vi "Retrieve Current Sample Data.vi"(8 "error in (no error)":errorcluster) -> (0 "error out":errorcluster, 1 "Last Sample":u32[](array[numeric]), 2 "Encoder Out":i32, 3 "Last Sample No.":u32, 4 "Partial Data":bool, 5 "nSamples":u32)   [LabVIEW 2015, in "Tool Module.lvlib"]
uses:
  Tool Module.lvlib
  ToolModGLOB.vi
  Tool Interface/Tool Interface.lvlib
  Tool Config/Tool Cfg.lvlib
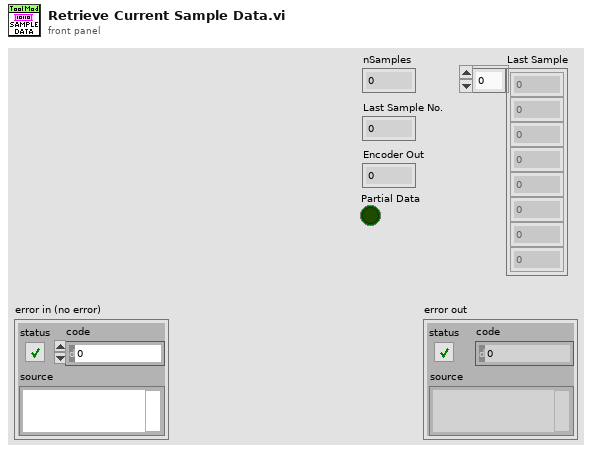
[diagram p1: front panel]
types:
  T1 = typedef "_Data Stream Fmt Params Cluster--typedef.ctl" = cluster{"Samples per Block":i32, "Raw Data Status Len":i32, "Fltr Data Status Len":i32}
  T2 = typedef "Tool Cfg.lvlib/_Tool Operation Config Cluster--typedef.ctl" = cluster{"Use Tool Cfg":bool, "Use Tool Cal":bool, "Fake Data?":bool, "Mode":i16, "Array Subset Length":i16, "nArrays to Read":i16, "Full Array Read Length":i16, "nSubarrays/Sensor":i16}
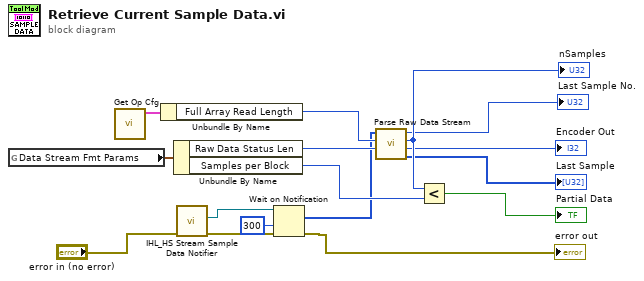
[diagram p0: block diagram]
diagram:
  n1 = global read "ToolModGLOB.vi" "Data Stream Fmt Params"() -> (w11:T1)
  n2 = call "Get Op Cfg.vi"() -> ("Tool Operation Config"=w13:T2)  [unwired: 11 in]
  n3 = Unbundle By Name(w13) -> ("Full Array Read Length"=w12:i16)
  n4 = Unbundle By Name(w11) -> ("Raw Data Status Len"=w10:i32, "Samples per Block"=w8:i32)
  n5 = call "IHL_HS Stream Sample Data Notifier.vi"("error in (no error)"="error in (no error)") -> ("error out"=w16:errorcluster, "Sample Data notifier out"=w15:refnum<notifier>)  [unwired: 9 in]
  n6 = Wait on Notification(notifier=w15, timeout in ms (-1)=300, error in (no error)=w16) -> (notification=w1:u32[], error out=→"error out":errorcluster)  [unwired: 1 in, 2 out]
  n7 = call "Parse Raw Data Stream.vi"("Status Hdr Length"=w10, "Pixel Array Length"=w12, "Sample Data Array"=w1) -> ("Last Sample"=→"Last Sample":u32[], "Encoder Out"=→"Encoder Out":i32, "nSamples"=w9:u32, "Last Sample No."=→"Last Sample No.":u32)  [unwired: 4 in, 1 out]
  "nSamples" <- w9
  n8 = Less?(x=w9, y=w8) -> (x < y?=→"Partial Data":bool)
